vi "Arm Pot Controller.vi"(1 "error in":errorcluster) -> (0 "error out":errorcluster)   [LabVIEW 2017]
uses:
  Global Simulated Arm Pot.vi
  <vilib>/addons/control/pid/pid.llb/PID (DBL).vi
  <vilib>/Rock Robotics/WPI/ThirdParty/Phoenix-LabVIEW/Motor Controller/Controls/CTRE_Phoenix_MotorControl_ControlMode.ctl
  <vilib>/addons/control/pid/NI_PID_pid.lvlib
panel:
  out "New Arm Position":dbl
  out "10% Scale Factor of Delta":dbl
  out "Arm Set Point - Arm Pot Value":dbl
  out "Waveform Chart":T1(graph)
  out "dt out (s)":dbl format="%.3f"
  out "Arm Pot Value":dbl
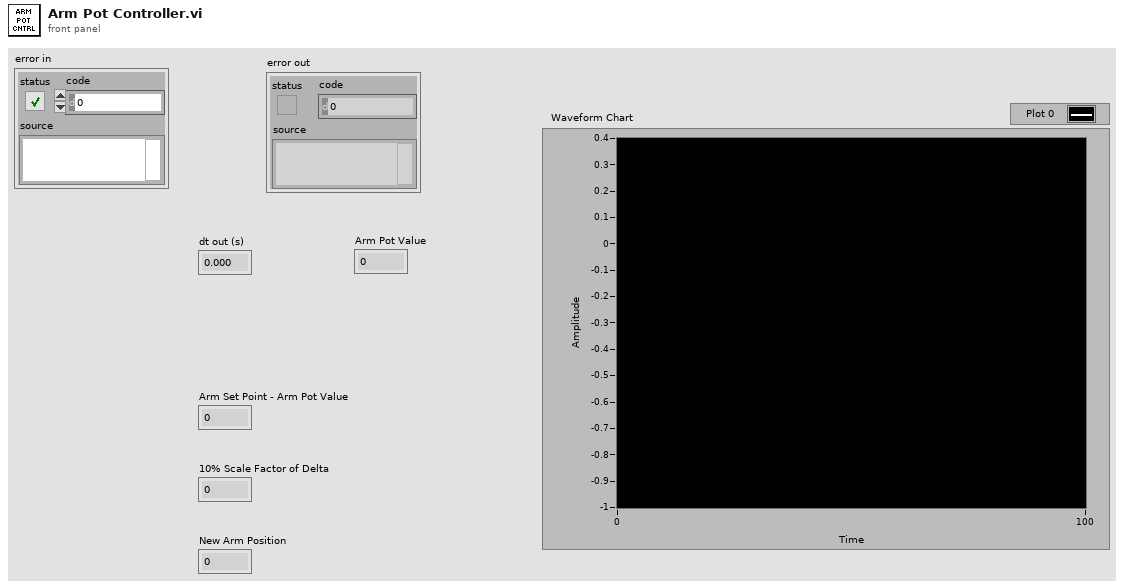
[diagram p1: front panel]
types:
  T1 = cluster{"Input":dbl, "output":dbl, "Simulated Arm Pot":dbl}
  T2 = cluster{"proportional gain (Kc)":dbl, "integral time (Ti, min)":dbl, "derivative time (Td, min)":dbl}
  T3 = typedef "WPI_PotentiometerDevRef.ctl" = cluster{"DevStatus":errorcluster, "Analog Channel":T4, "Invert Output":bool}
  T4 = typedef "FPGA_AIChannel.ctl" = enum8{"AI 0", "AI 1", "AI 2", "AI 3", "AI MXP 0", "AI MXP 1", "AI MXP 2", "AI MXP 3", "Invalid"}
  T5 = cluster{"Arm Setpoint":dbl, "Simulated Arm Pot":dbl, "Simulated Arm Pot":dbl}
  T6 = typedef "CTRE_Phoenix_MotorControl_ControlMode.ctl" = u16
  T7 = typedef "WPI_MotorControlDeviceRef.ctl" = cluster{"DeviceStatus":errorcluster, "Type":T8, "PWM":cluster{"PWM Channel":T9, "DeadBand":T10}, "CAN":cluster{"Device Number":u8, "SetOutput VI Ref":variant, "GetOutput VI Ref":variant, "Enable VI Ref":variant, "Disable VI Ref":variant, "Data":variant}, "Invert":bool, "DIO PWM":cluster{"PWM \"Enable\" Channel":T9, "DIOChannel":T11, "PWM Rate":dbl}}
  T8 = typedef "WPI_MotorControlType.ctl" = enum16{"PWM", "CAN", "DIO PWM"}
  T9 = typedef "FPGA_DIOPWMChannel.ctl" = enum8{"PWM 0", "PWM 1", "PWM 2", "PWM 3", "PWM 4", "PWM 5", "PWM 6", "PWM 7", "PWM 8", "PWM 9", "PWM MXP 0", "PWM MXP 1", "PWM MXP 2", "PWM MXP 3", "PWM MXP 4", "PWM MXP 5", "PWM MXP 6", "PWM MXP 7", "PWM MXP 8", "PWM MXP 9", "Invalid"}
  T10 = typedef "WPI_PWMDeadband.ctl" = cluster{"Name":string, "maxPositivePwm":i32, "minPositivePwm":i32, "centerPwm":i32, "maxNegativePwm":i32, "minNegativePwm":i32, "angularRange":u16}
  T11 = typedef "FPGA_DIOChannel.ctl" = enum8{"DIO 0", "DIO 1", "DIO 2", "DIO 3", "DIO 4", "DIO 5", "DIO 6", "DIO 7", "DIO 8", "DIO 9", "DIO MXP 0", "DIO MXP 1", "DIO MXP 2", "DIO MXP 3", "DIO MXP 4", "DIO MXP 5", "DIO MXP 6", "DIO MXP 7", "DIO MXP 8", "DIO MXP 9", "DIO MXP 10", "DIO MXP 11", "DIO MXP 12", "DIO MXP 13", "DIO MXP 14", "DIO MXP 15", "SPI Port CS1", "SPI Port CS2", "SPI Port CS3", "SPI Port MISO", "SPI Port MOSI", "Invalid"}
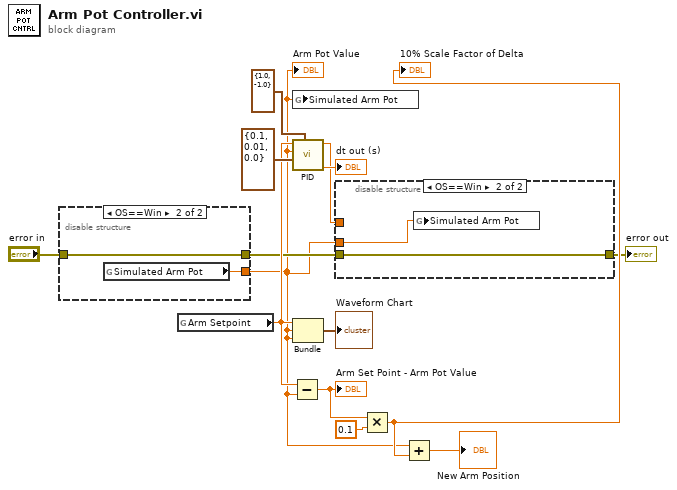
[diagram p0: block diagram]
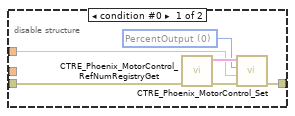
[diagram p2: hidden frame]
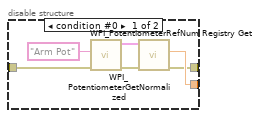
[diagram p3: hidden frame]
diagram:
  n1 = disable-structure shown="OS==Win" {
    disable-tunnel: "error in" -> [w18 w22]
    disable-tunnel: [w19 w21] -> w1
    disable-tunnel: [w16 w22] -> w3
    frame condition #0 {
      n2 = call <vilib>:"WPI_PotentiometerRefNum Registry Get.vi"("error in (no error)"=w18, "refnum name"="Arm Pot") -> ("error out"=w17:errorcluster, "PotDevRef"=w20:T3)  [unwired: 8 in]
      n3 = call <vilib>:"WPI_PotentiometerGetNormalized.vi"("error in"=w17, "PotDevRef"=w20) -> ("error out"=w16:errorcluster, "Normalized Value"=w19:dbl)  [unwired: 7 in, 1 out]
    }
    frame condition #1 (active) {
      n4 = global read "Global Simulated Arm Pot.vi" "Simulated Arm Pot"() -> (w21:dbl)
    }
  }
  "Arm Pot Value" <- w1
  n5 = global read "Global Simulated Arm Pot.vi" "Arm Setpoint"() -> (w5:dbl)
  n6 = Subtract(x=w5, y=w1) -> (x-y=w9:dbl)
  "Arm Set Point - Arm Pot Value" <- w9
  n7 = global write "Global Simulated Arm Pot.vi" "Simulated Arm Pot"(w1) -> ()
  n8 = call-poly <vilib>:"PID.vi"("output range"=cluster{"output high":dbl, "output low":dbl} {"output high"=1.0, "output low"=-1.0}, "PID gains"=T2 {"proportional gain (Kc)"=0.1, "integral time (Ti, min)"=0.01, "derivative time (Td, min)"=0.0}, "process variable"=w1, "setpoint"=w5) -> ("dt out (s)"=→"dt out (s)":dbl, "output"=w4:dbl)  [unwired: 6 in]
  n9 = Bundle("Arm Setpoint"=w5, "Simulated Arm Pot"=w1, "Simulated Arm Pot"=w1) -> (→"Waveform Chart":T5)  [unwired: 1 in]
  n10 = disable-structure shown="OS==Win" {
    disable-tunnel: [w25 w30] -> w2
    disable-tunnel: w4 -> [w24 _]
    disable-tunnel: w3 -> [w23 w30]
    disable-tunnel: w1 -> [_ w29]
    frame condition #0 {
      w27 = T6 0 items=["PercentOutput"=0, "Position"=1, "Velocity"=2, "Current"=3, "Follower"=5, "MotionProfile"=6, "MotionMagic"=7, "MotionMagicArc"=8, "MotionProfileArc"=10, "Disabled"=15] ("Control Mode")
      n11 = call <vilib>:"CTRE_Phoenix_MotorControl_RefNumRegistryGet.vi"("error in (no error)"=w23) -> ("error out"=w26:errorcluster, "PhoenixMotorControlDevRef"=w28:T7)  [unwired: 9 in]
      n12 = call <vilib>:"CTRE_Phoenix_MotorControl_Set.vi"("error in (no error)"=w26, "Output"=w24, "Control Mode"=w27, "PhoenixMotorControlDevRef"=w28) -> ("error out"=w25:errorcluster)  [unwired: 6 in, 1 out]
    }
    frame condition #1 (active) {
      n13 = global write "Global Simulated Arm Pot.vi" "Simulated Arm Pot"(w29) -> ()
    }
  }
  "error out" <- w2
  n14 = Multiply(x=w9, y=0.1) -> (x*y=w7:dbl)
  "10% Scale Factor of Delta" <- w7
  n15 = Add(x=w1, y=w7) -> (x+y=→"New Arm Position":dbl)
